vi "Handle Error Handler Errors.vi"(8 "error in (no error)":errorcluster, 11 "Process In":refnum<class "Process.lvclass">) -> (0 "error out":errorcluster, 3 "Process Out":refnum<class "Process.lvclass">)   [LabVIEW 2020, in "Error Handler.lvclass"]
uses:
  Error Handler.lvclass
  Process/Process.lvclass
  Community/TypeDefs/Error Message Data.ctl
  Process/Process.lvclass/Process.ctl
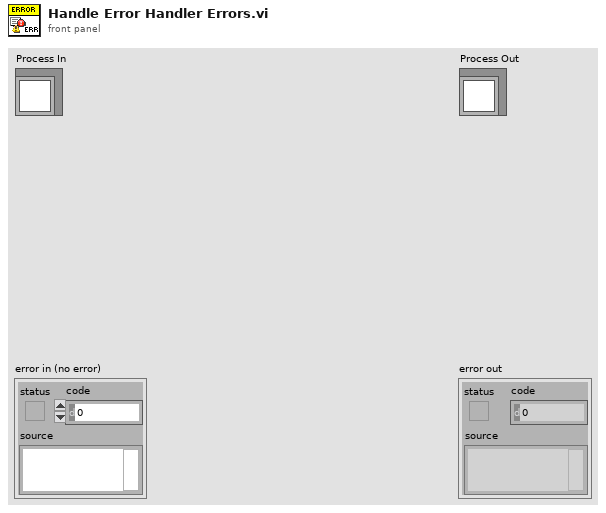
[diagram p1: front panel]
types:
  T1 = typedef "Error Handler.lvclass/Error Message Data.ctl" = cluster{"Error Type":string, "Location":string, "Error":errorcluster}
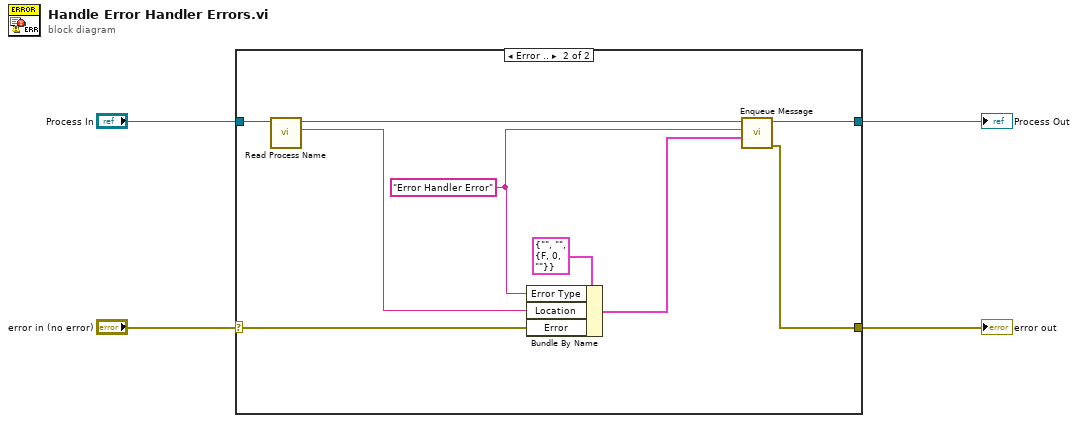
[diagram p0: block diagram]
diagram:
  n1 = case shown="Error .." "error in (no error)" {
    selector: "error in (no error)" -> [w6 w11]
    tunnel: "Process In" -> [w5 w13]
    tunnel: [w5 w10] -> w3
    tunnel: [w6 w9] -> w1
    frame No Error {
    }
    frame Error {
      w7 = "Error Handler Error" ("Error Type")
      n2 = call "Read Process Name.vi"("Process In"=w13) -> ("Process Name"=w12:string, "Process Out"=w14:refnum<class "Process.lvclass">)  [unwired: 9 in]
      n3 = Bundle By Name(cluster=T1 {"Error Type"="", "Location"="", "Error"={"status"=FALSE, "code"=0, "source"=""}} ("Error Message Data"), "Error Type"=w7, "Location"=w12, "Error"=w11) -> (w8:T1)
      n4 = call "Enqueue Message.vi"("Message Data"=w8, "Message"=w7, "Process In"=w14) -> ("error out"=w9:errorcluster, "Process Out"=w10:refnum<class "Process.lvclass">)  [unwired: 7 in]
    }
  }
  "error out" <- w1
  "Process Out" <- w3
